vi "CelsiusToFarhenheit.vi"() -> ()   [LabVIEW 2019]
panel:
  out "Temp (F)":dbl
  in  "Temp (C)":dbl
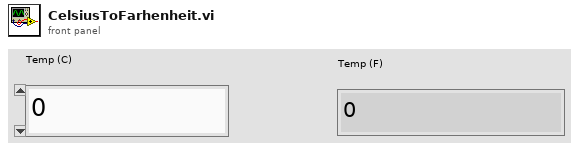
[diagram p1: front panel]
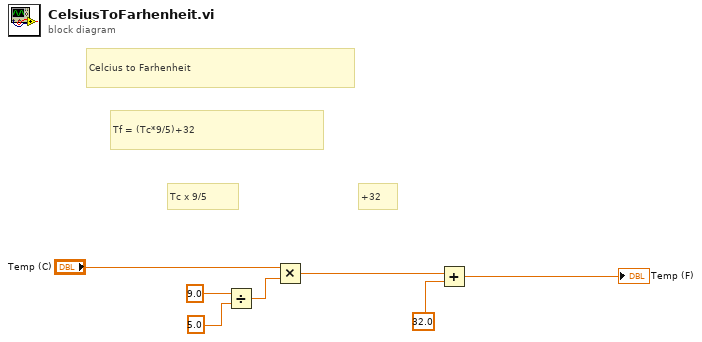
[diagram p0: block diagram]
diagram:
  # "+32"
  # "Tc x 9/5"
  # "Tf = (Tc*9/5)+32"
  # "Celcius to Farhenheit"
  n1 = Divide(x=9.0, y=5.0) -> (x/y=w4:dbl)
  n2 = Multiply(x="Temp (C)", y=w4) -> (x*y=w3:dbl)
  n3 = Add(x=w3, y=32.0) -> (x+y=→"Temp (F)":dbl)
